vi "ValueUpperLowerReadings.vi"(0 "Target Value":dbl, 1 "Lower X Error Value (type -0.01 for neg 10mV)":dbl, 2 "Upper X Error Value (type 0.01 for pos 10mV)":dbl, 3 "X Data (sorted)":dbl[](array[numeric]), 4 "Y Data":dbl[](array[numeric])) -> (5 "Interpolated Result":dbl, 6 "Error":dbl)   [LabVIEW 2017]
doc: "Takes in an ascending ordered X array and a Y array and interpolates the value. Given an upper error and lower value, it will interpolate the corresponding upper and lower Y errors."
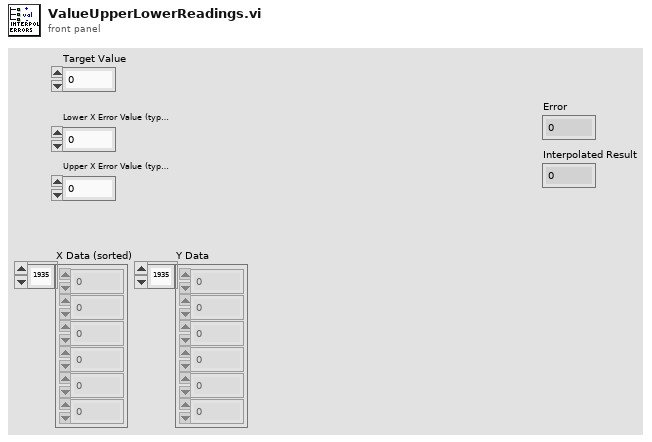
[diagram p1: front panel]
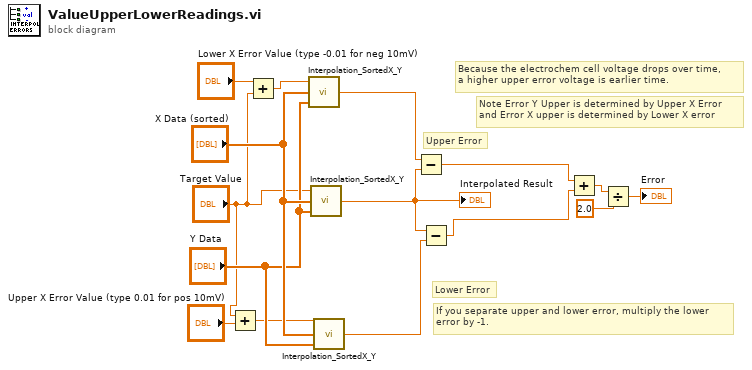
[diagram p0: block diagram]
diagram:
  # "If you separate upper and lower error, multiply the lower\nerror by -1."
  # "Lower Error"
  # "Upper Error"
  # "Note Error Y Upper is determined by Upper X Error\nand Error X upper is determined by Lower X error"
  # "Because the electrochem cell voltage drops over time,\na higher upper error voltage is earlier time."
  n1 = Add(x="Target Value", y="Upper X Error Value (type 0.01 for pos 10mV)") -> (x+y=w8:dbl)
  n2 = Add(x="Lower X Error Value (type -0.01 for neg 10mV)", y="Target Value") -> (x+y=w6:dbl)
  n3 = call "Interpolation_SortedX_Y.vi"("Y Data"="Y Data", "X Data (sorted)"="X Data (sorted)", "Target X (threshold)"=w6) -> ("Interpolated Results"=w13:dbl)
  n4 = call "Interpolation_SortedX_Y.vi"("Y Data"="Y Data", "X Data (sorted)"="X Data (sorted)", "Target X (threshold)"="Target Value") -> ("Interpolated Results"=w12:dbl)
  "Interpolated Result" <- w12
  n5 = call "Interpolation_SortedX_Y.vi"("Y Data"="Y Data", "X Data (sorted)"="X Data (sorted)", "Target X (threshold)"=w8) -> ("Interpolated Results"=w11:dbl)
  n6 = Subtract(x=w13, y=w12) -> (x-y=w5:dbl)
  n7 = Subtract(x=w12, y=w11) -> (x-y=w4:dbl)
  n8 = Add(x=w5, y=w4) -> (x+y=w3:dbl)
  n9 = Divide(x=w3, y=2.0) -> (x/y=→"Error":dbl)
